vi "FormulaScript.vi"() -> ()   [LabVIEW 2020]
panel:
  out "Hipotenusa":dbl
  in  "cateto b":dbl
  in  "cateto a":dbl
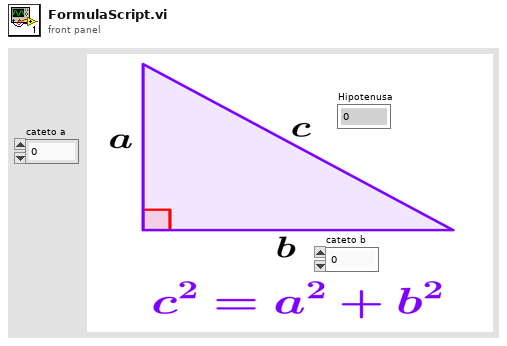
[diagram p1: front panel]
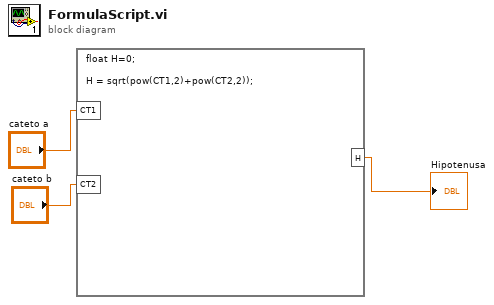
[diagram p0: block diagram]
diagram:
  n1 = formula code="float H=0;\n\nH = sqrt(pow(CT1,2)+pow(CT2,2));"("CT1"="cateto a", "CT2"="cateto b") -> ("H"=→"Hipotenusa":dbl)
